vi "Do Coordinate.vi"(10 "Player ID":i32, 11 "TeamEffort in":refnum<class "TeamEffort.lvclass">) -> (1 "Coordinated Move?":bool, 2 "Calc Master?":bool, 3 "TeamEffort out":refnum<class "TeamEffort.lvclass">)   [LabVIEW 2015, in "TeamEffort.lvclass"]
uses:
  TeamEffort.lvclass
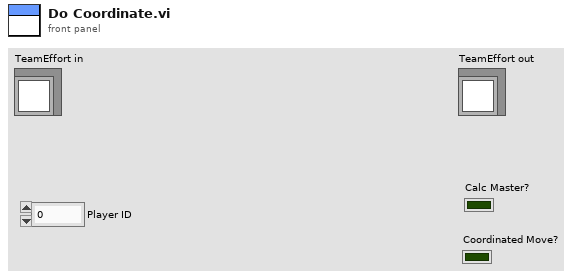
[diagram p1: front panel]
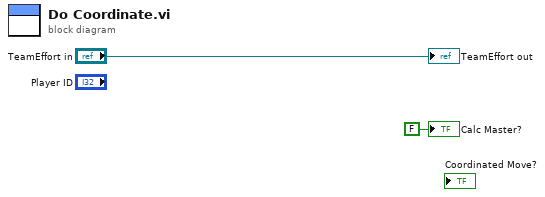
[diagram p0: block diagram]
diagram:
  "TeamEffort out" <- "TeamEffort in"
  "Calc Master?" <- FALSE ("Calc Master?")
